vi "Static Demo 2.vi"() -> ()   [LabVIEW 2020]
uses:
  <extravilib>/Connections/Connection-t'Function Generator.lvlib-Shape.ctl'.lvclass
  <extravilib>/Connections/Connection-dbl.lvclass
  <extravilib>/Connections/Connection-c(dbl,dbl,a[.](cdb)).lvclass
  FlexBlocks/Shape.ctl
  Workers/Function Generator/Function Generator.lvlib
panel:
  out "Latest":cluster{"t0":dbl, "dt":dbl, "y":cdb[]}
  out "Graph":cluster{"t0":dbl, "dt":dbl, "y":dbl[]}(graph)
  in  "stop":bool
  in  "Offset":dbl
  in  "Phase":dbl
  in  "Amplitude":dbl
  in  "Frequency":dbl
  in  "Shape":T1
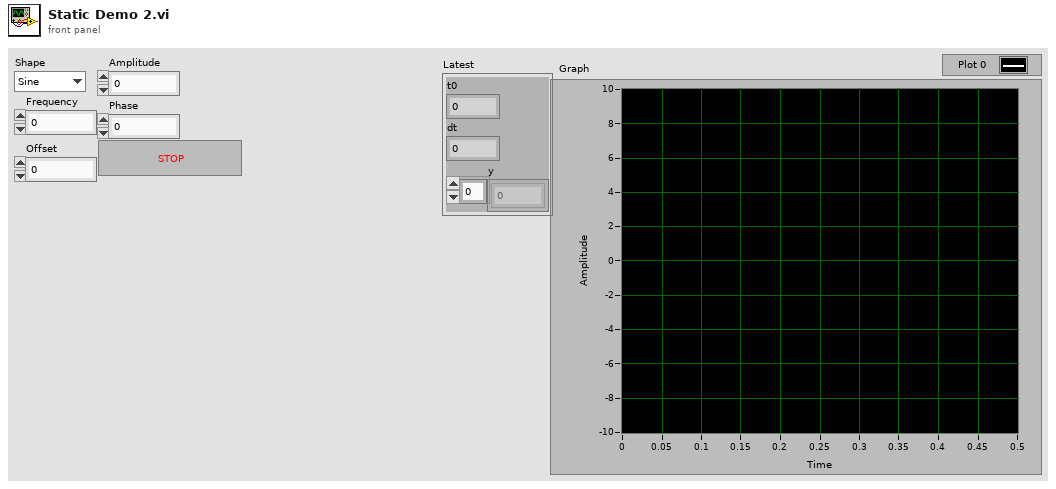
[diagram p1: front panel]
types:
  T1 = typedef "Function Generator.lvlib/Shape.ctl" = enum16{"Sine", "Square", "Triangle", "Saw"}
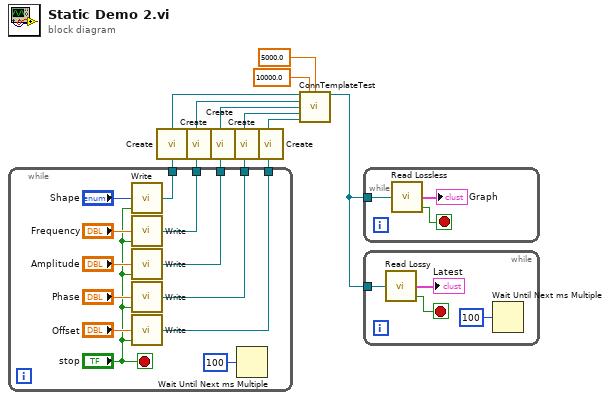
[diagram p0: block diagram]
diagram:
  n1 = call <extravilib>:"Create.vi"() -> ("Connection"=w8:refnum<class "Connection-t'Function Generator.lvlib-Shape.ctl'.lvclass">)
  n2 = call <extravilib>:"Create.vi"() -> ("Connection"=w7:refnum<class "Connection-dbl.lvclass">)
  n3 = call <extravilib>:"Create.vi"() -> ("Connection"=w6:refnum<class "Connection-dbl.lvclass">)
  n4 = call <extravilib>:"Create.vi"() -> ("Connection"=w5:refnum<class "Connection-dbl.lvclass">)
  n5 = call <extravilib>:"Create.vi"() -> ("Connection"=w4:refnum<class "Connection-dbl.lvclass">)
  n6 = while {
    tunnel: w8 -> [w19]
    tunnel: w7 -> [w18]
    tunnel: w6 -> [w17]
    tunnel: w5 -> [w16]
    tunnel: w4 -> [w15]
    stop <- "stop" stop-if-true
    n7 = call <extravilib>:"Write.vi"("Connection"=w19, "Close? (F)"="stop", "Element"="Shape") -> ()  [unwired: 1 in, 2 out]
    n8 = call <extravilib>:"Write.vi"("Connection"=w18, "Close? (F)"="stop", "Element"="Frequency") -> ()  [unwired: 1 in, 2 out]
    n9 = call <extravilib>:"Write.vi"("Connection"=w17, "Close? (F)"="stop", "Element"="Amplitude") -> ()  [unwired: 1 in, 2 out]
    n10 = call <extravilib>:"Write.vi"("Connection"=w16, "Close? (F)"="stop", "Element"="Phase") -> ()  [unwired: 1 in, 2 out]
    n11 = call <extravilib>:"Write.vi"("Connection"=w15, "Close? (F)"="stop", "Element"="Offset") -> ()  [unwired: 1 in, 2 out]
    n12 = Wait Until Next ms Multiple(millisecond multiple=u32 100) -> ()  [unwired: 1 out]
  }
  n13 = call "ConnTemplateTest.vi"("Shape"=w8, "Sample Rate"=10000.0, "Sample Count"=5000.0 ("Sample Rate"), "Frequency"=w7, "Amplitude"=w6, "Phase"=w5, "Offset"=w4) -> ("Out"=w3:refnum<class "Connection-c(dbl,dbl,a[.](cdb)).lvclass">)  [unwired: 8 in]
  n14 = while {
    tunnel: w3 -> [w23]
    stop <- w21 stop-if-true
    n15 = call <extravilib>:"Read Lossless.vi"("Connection"=w23) -> ("Closed?"=w21:bool, "Element"=→"Graph":cluster{"t0":dbl, "dt":dbl, "y":cdb[]})  [unwired: 2 in, 1 out]
  }
  n16 = while {
    tunnel: w3 -> [w27]
    stop <- w25 stop-if-true
    n17 = call <extravilib>:"Read Lossy.vi"("Connection"=w27) -> ("Closed?"=w25:bool, "Element"=→"Latest":cluster{"t0":dbl, "dt":dbl, "y":cdb[]})  [unwired: 2 in, 1 out]
    n18 = Wait Until Next ms Multiple(millisecond multiple=u32 100) -> ()  [unwired: 1 out]
  }
